vi "Var Tools Speed.vi"() -> ()   [LabVIEW 2017]
uses:
  f7c238da-8fbc-4fee-af8f-df2d97f3cdd7.vi
  Variant to JSON Text.vi
  <vilib>/Utility/VariantDataType/VariantType.lvlib
  <vilib>/Utility/Data Type/NI_Data Type.lvlib
panel:
  out "Array":string[](array[string])
  out "match substring":string
  out "x/y":dbl format="%#_6p"
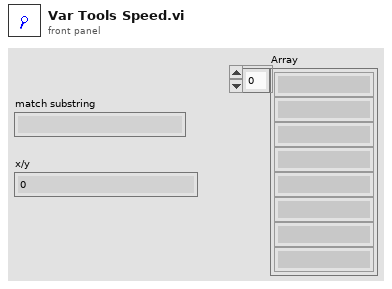
[diagram p1: front panel]
types:
  T1 = typedef "VariantType.lvlib/Type.ctl" = enum8{"Invalid Type", "Void", "I8", "I16", "I32", "I64", "U8", "U16", "U32", "U64", "Single Float", "Double Float", "Extended Float", "Single Complex", "Double Complex", "Extended Complex", "Enum U8", "Enum U16", "Enum U32", "Enum U64", "Single Float With Unit", "Double Float With Unit", "Extended Float With Unit", "Single Complex with Unit", "Double Complex with Unit", "Extended Complex with Unit", "Boolean", "String", "Path", "Picture", "Tag", "Array", "Cluster", "Variant", "LV Variant", "Waveform", "Timestamp", "Digital Waveform", "Digital Data", "ExpressData", "Refnum", "External Data", "VI", "Poly VI", "LabVIEW Class Instance", "Fixed Point"}
  T2 = typedef "NI_Data Type.lvlib/Data Type.ctl" = enum8{"Invalid Type", "Void", "I8", "I16", "I32", "I64", "U8", "U16", "U32", "U64", "Single Float", "Double Float", "Extended Float", "Single Complex", "Double Complex", "Extended Complex", "Enum U8", "Enum U16", "Enum U32", "Enum U64", "Single Float With Unit", "Double Float With Unit", "Extended Float With Unit", "Single Complex with Unit", "Double Complex with Unit", "Extended Complex with Unit", "Boolean", "String", "Path", "Picture", "Tag", "Array", "Cluster", "Variant", "LV Variant", "Waveform", "Timestamp", "Digital Waveform", "Digital Data", "ExpressData", "Refnum", "External Data", "VI", "Poly VI", "LabVIEW Class Instance", "Fixed Point"}
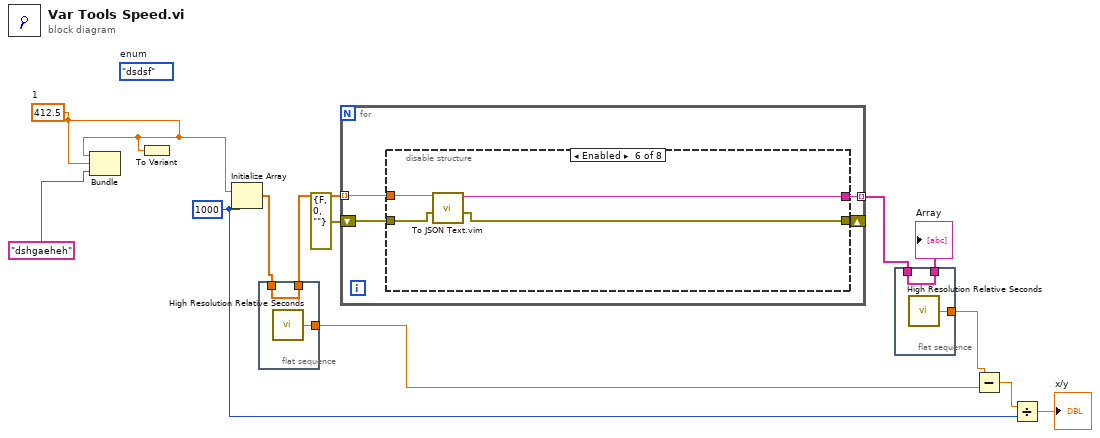
[diagram p0: block diagram]
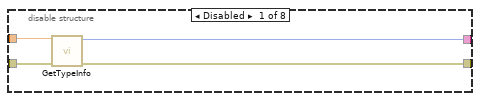
[diagram p2: hidden frame]
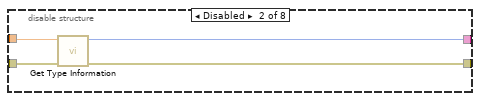
[diagram p3: hidden frame]
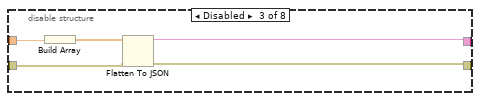
[diagram p4: hidden frame]
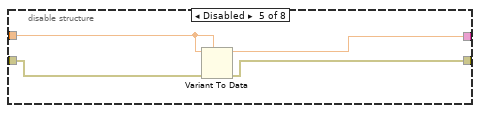
[diagram p6: hidden frame]
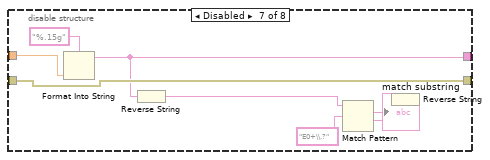
[diagram p7: hidden frame]
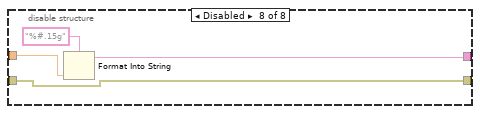
[diagram p8: hidden frame]
diagram:
  w2 = 412.5  # 1
  (unwired) enum16{"dsdsf", "sdagads", "gsd", "gsgvdsg"}."dsdsf"  # enum
  w5 = 1000 ("dimension size")
  n1 = Bundle("1"=w2, "1"=w2, "dshgaeheh") -> ()  [unwired: 1 in, 1 out]
  n2 = To Variant(anything=w2) -> ()  [unwired: 1 out]
  n3 = Initialize Array(w2, w5) -> (w11:dbl[])
  n4 = flat-sequence {
    tunnel: w11 -> [w14]
    tunnel: [w14] -> w10
    tunnel: [w13] -> w7
    frame #0 {
      n5 = call <vilib>:"High Resolution Relative Seconds.vi"() -> ("relative seconds"=w13:dbl)
    }
  }
  n6 = for {
    tunnel: w10 -> [w18] mode=indexing
    tunnel: [w17] -> w9 mode=indexing
    shift-right: [w16] -> _
    shift-left: errorcluster {"status"=FALSE, "code"=0, "source"=""} ("error out") -> [w15]
    n7 = disable-structure shown="Enabled" {
      disable-tunnel: w18 -> [w22 w26 w28 w32 w37 w41 w49 w53]
      disable-tunnel: [w21 w25 w30 w32 w34 w40 w43 w52] -> w17
      disable-tunnel: [w20 w23 w29 w33 w35 w38 w48 w51] -> w16
      disable-tunnel: w15 -> [w19 w24 w31 w33 w36 w39 w48 w51]
      frame Disabled {
        n8 = call <vilib>:"GetTypeInfo.vi"("error in (no error)"=w19, "Variant"=w22) -> ("error out"=w20:errorcluster, "Type Enum"=w21:T1)  [unwired: 5 in, 3 out]
      }
      frame Disabled {
        n9 = call <vilib>:"Get Type Information.vi"("error in (no error)"=w24, "Variant"=w26) -> ("error out"=w23:errorcluster, "Type"=w25:T2)  [unwired: 5 in, 3 out]
      }
      frame Disabled {
        n10 = Build Array(w28) -> (w27:dbl[])
        n11 = Flatten To JSON(anything=w27, error in (no error)=w31) -> (JSON string=w30:string, 11:w29:errorcluster)  [unwired: 1 in]
      }
      frame Disabled {
      }
      frame Disabled {
        n12 = Variant To Data(error in=w36, type=w37, Variant=w37) -> (data=w34:dbl, error out=w35:errorcluster)
      }
      frame Enabled {
        n13 = call "To JSON Text.vim"("error in (no error)"=w39, "Anything"=w41) -> ("error out"=w38:errorcluster, "<JSON>"=w40:string)  [unwired: 8 in]
      }
      frame Disabled {
        n14 = Format Into String(format string="%.15g", w49) -> (resulting string=w43:string)  [unwired: 2 in, 1 out]
        n15 = Reverse String(1:w43) -> (0:w45:string)
        n16 = Match Pattern(string=w45, regular expression="E0+\\.?") -> (match substring=→"match substring":string, after substring=w44:string)  [unwired: 1 in, 2 out]
        n17 = Reverse String(1:w44) -> ()  [unwired: 1 out]
      }
      frame Disabled {
        n18 = Format Into String(format string="%#.15g", w53) -> (resulting string=w52:string)  [unwired: 2 in, 1 out]
      }
    }
  }
  n19 = flat-sequence {
    tunnel: w9 -> [w55]
    tunnel: [w55] -> w1
    tunnel: [w54] -> w8
    frame #0 {
      n20 = call <vilib>:"High Resolution Relative Seconds.vi"() -> ("relative seconds"=w54:dbl)
    }
  }
  n21 = Subtract(x=w8, y=w7) -> (x-y=w6:dbl)
  n22 = Divide(x=w6, y=w5) -> (x/y=→"x/y":dbl)
  "Array" <- w1
